vi "Audio_Transformation_Setted_Frequency_v003.vi"() -> ()   [LabVIEW 2019]
uses:
  <vilib>/sound2/lvsound2.llb/Sound Data Format.ctl
  <vilib>/sound2/lvsound2.llb/Sound Input Read (DBL).vi
  <vilib>/addons/Time Frequency Analysis/Transform.llb/TFA Online Gabor Transform (Real).vi
  <vilib>/addons/Time Frequency Analysis/Transform.llb/TFA Online Gabor Expansion (Real).vi
  <vilib>/addons/_Advanced Signal Processing/NI_AdvSigProcTFA.lvlib
panel:
  out "max index(es) 2":i32
  out "max value 2":dbl
  out "Waveform Chart 2":dbl[](graph)
  out "Enhanced Speech":dbl[](graph)
  in  "Enhance?":bool
  in  "Attenuation factor":dbl
  in  "Noise level":dbl
  out "Enhanced Gabor Coefficients":dbl[][](graph)
  out "Noise Speech":dbl[](graph)
  out "u(t)":dbl(graph)
  out "V(t)":dbl(graph)
  in  "Address selector":i32[](array[numeric])
  in  "Neuron Type":T1(ring)
  out "max index(es)":i32
  out "max value":dbl
  out "Waveform Chart":dbl[](graph)
  out "Magnitude of Gabor Coefficients":dbl[][](graph)
  in  "Stop":bool
  # "Step two : Graph of the amplitude of the Gabor coefficient of the different bins"
  # "Step one: Sound recorded from the computer"
  # "Step three : Spike Response of the neuron"
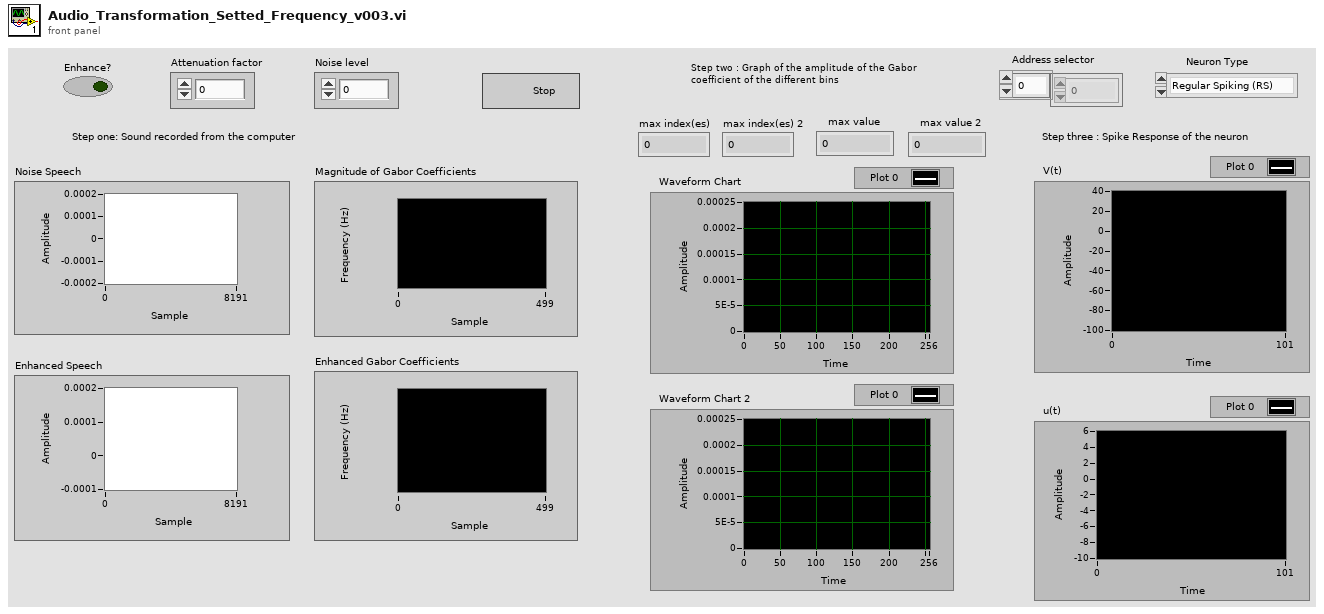
[diagram p1: front panel]
types:
  T1 = enum16{"Regular Spiking (RS)", "Intrinsically Bursting (IB)", "Chattering (CH)", "Fast Spiking (FS)", "Thalamo-Cortical 1 (TC1)", "Thalamo-Cortical 2 (TC2)", "Resonator (RZ)", "Low-Threshold Spiking (LTS)"}
  T2 = typedef "Sound Data Format.ctl" = cluster{"sample rate (S/s)":dbl, "number of channels":i32, "bits per sample":i32}
  T3 = typedef "Sound Input Task ID.ctl" = u32
  T4 = cluster{"analysis window":dbl[], "dM (time steps)":i32, "N (frequency bins)":i32}
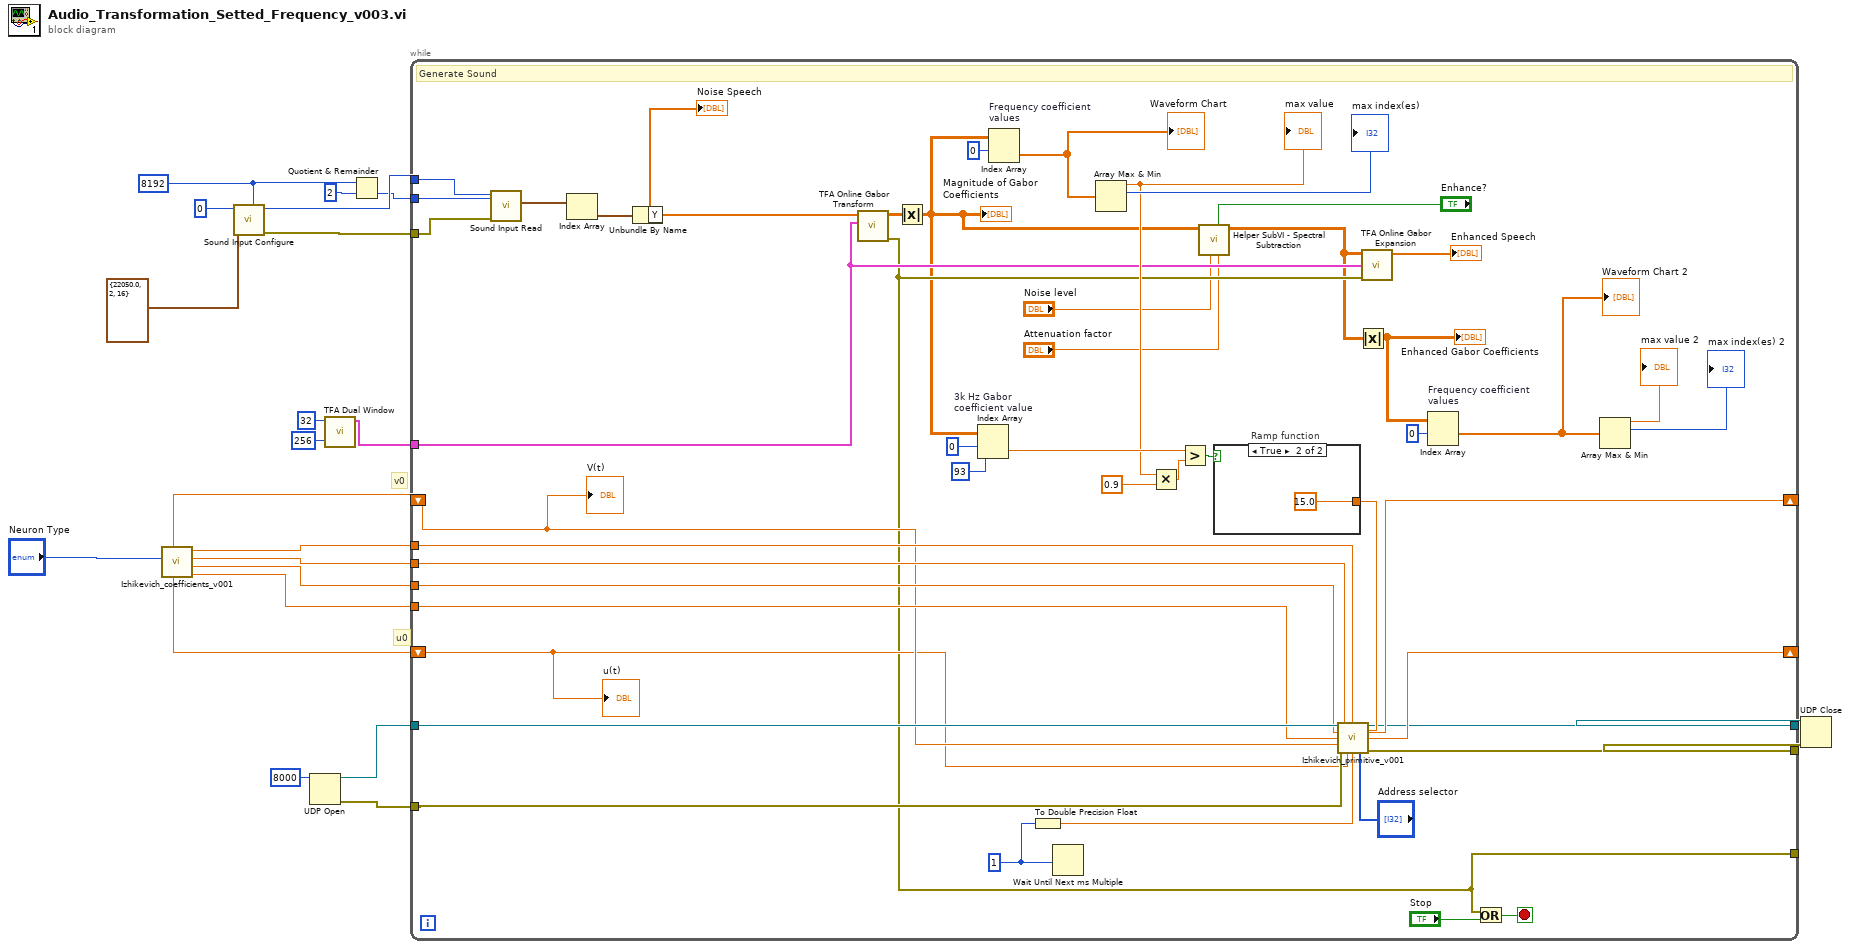
[diagram p0: block diagram]
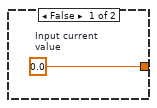
[diagram p2: hidden frame]
diagram:
  w2 = 8192 ("number of samples/ch")
  # "u0"
  # "v0"
  n1 = call "Izhikevich_coefficients_v001.vi"("Neuron Type"="Neuron Type") -> ("d"=w13:dbl, "c"=w14:dbl, "b"=w15:dbl, "a"=w16:dbl, "u0"=w17:dbl, "v0"=w18:dbl)  [unwired: 3 in]
  n2 = call <vilib>:"Sound Input Configure.vi"("number of samples/ch"=w2, "sound format"=T2 {"sample rate (S/s)"=22050.0, "number of channels"=2, "bits per sample"=16}, "device ID"=u32 0) -> ("error out"=w5:errorcluster, "task ID"=w6:T3)  [unwired: 7 in]
  n3 = UDP Open(11:u16 8000 ("port")) -> (port=w11:refnum<k16>, 0:w10:errorcluster)  [unwired: 4 in, 1 out]
  n4 = call <vilib>:"TFA Dual Window.vi"("N (frequency bins)"=256, "dM (time steps)"=32) -> ("analysis info"=w20:T4)  [unwired: 7 in, 2 out]
  n5 = Quotient & Remainder(x=w2, y=2) -> (floor(x/y)=w4:i32)  [unwired: 1 out]
  n6 = while {
    tunnel: [w34] -> _
    tunnel: w20 -> [w35]
    shift-right: [w50] -> _
    shift-left: w18 -> [w46]
    shift-right: [w49] -> _
    shift-left: w17 -> [w45]
    tunnel: w16 -> [w59]
    tunnel: w15 -> [w58]
    tunnel: w14 -> [w56]
    tunnel: w13 -> [w55]
    tunnel: w11 -> [w57]
    tunnel: w10 -> [w54]
    tunnel: [w48] -> w9
    tunnel: [w47] -> w8
    tunnel: w6 -> [w43]
    tunnel: w5 -> [w42]
    tunnel: w4 -> [w44]
    stop <- w69 stop-if-true
    w52 = u32 1 ("millisecond multiple")
    # "Generate Sound"
    n7 = call-poly <vilib>:"Sound Input Read.vi"("number of samples/ch"=w44, "error in (no error)"=w42, "task ID"=w43) -> ("data"=w40:waveform(dbl)[])  [unwired: 6 in, 2 out]
    n8 = Index Array(array=w40) -> (element=w41:waveform(dbl))  [unwired: 1 in]
    n9 = Unbundle By Name(w41) -> ("Y"=w39:dbl[])
    "Noise Speech" <- w39
    n10 = call-poly <vilib>:"TFA Online Gabor Transform.vi"("transform info"=w35, "signal"=w39) -> ("error out"=w34:errorcluster, "Gabor coef"=w68:cdb[][])  [unwired: 7 in, 1 out]
    n11 = Absolute Value(x=w68) -> (abs(x)=w33:dbl[][])
    "Magnitude of Gabor Coefficients" <- w33
    n12 = Index Array "3k Hz Gabor \ncoefficient value"(array=w33, index (row)=0, index (col)=93 ("disabled index (col)")) -> (element=w62:dbl)
    n13 = Index Array "Frequency coefficient \nvalues"(array=w33, index (row)=0) -> (element=w66:dbl[])  [unwired: 1 in]
    "Waveform Chart" <- w66
    n14 = To Double Precision Float(number=w52) -> (double precision float=w51:dbl)
    n15 = Wait Until Next ms Multiple(millisecond multiple=w52) -> ()  [unwired: 1 out]
    n16 = Array Max & Min(array=w66) -> (max value=w36:dbl, max index (indices)=→"max index(es)":i32)  [unwired: 2 out]
    "max value" <- w36
    n17 = Multiply(x=w36, y=0.9) -> (x*y=w38:dbl)
    n18 = Greater?(x=w62, y=w38) -> (0:w61:bool)
    n19 = call "Helper SubVI - Spectral Subtraction.vi"("attenuation factor"="Attenuation factor", "Enhance?"="Enhance?", "noise level"="Noise level", "Gabor coefficients in"=w33) -> ("Gabor coefficients out"=w28:cdb[][])  [unwired: 1 in, 6 out]
    n20 = case "Ramp function" shown="True" w61 {
      tunnel: [w71 15.0 ("Input current \nvalue")] -> w60
      frame False {
        w71 = 0.0  # Input current  value
      }
      frame True {
      }
    }
    n21 = call "Izhikevich_primitive_v001.vi"("UDP Network Connection in"=w57, "b"=w58, "a"=w59, "I"=w60, "c"=w56, "d"=w55, "v(t)"=w46, "error in (no error)"=w54, "u(t)"=w45, "Numeric"=w51, "Address selector"="Address selector") -> ("UDP Network Connection out"=w47:refnum<k16>, "v(t+dt)"=w50:dbl, "u(t+dt)"=w49:dbl, "error out"=w48:errorcluster)  [unwired: 1 in]
    n22 = Absolute Value(x=w28) -> (abs(x)=w26:dbl[][])
    "Enhanced Gabor Coefficients" <- w26
    n23 = call-poly <vilib>:"TFA Online Gabor Expansion.vi"("error in (no error)"=w34, "expansion info"=w35, "Gabor coef"=w28) -> ("signal"=→"Enhanced Speech":dbl[])  [unwired: 1 in, 7 out]
    n24 = Index Array "Frequency coefficient \nvalues"(array=w26, index (row)=0) -> (element=w23:dbl[])  [unwired: 1 in]
    "Waveform Chart 2" <- w23
    n25 = Or(x=w34, y="Stop") -> (x .or. y?=w69:bool)
    n26 = Array Max & Min(array=w23) -> (max value=→"max value 2":dbl, max index (indices)=→"max index(es) 2":i32)  [unwired: 2 out]
    "V(t)" <- w46
    "u(t)" <- w45
  }
  n27 = UDP Close(connection ID=w8, 8:w9) -> ()  [unwired: 2 out]
